vi "Create Data Clusters for Types.vi"(6 "Enum parameters":T1[](array[typedef]), 7 "Message parameters":T2[](array[typedef]), 8 "error in (no error)":errorcluster, 11 "Library in":refnum<vi>) -> (0 "error out":errorcluster, 3 "Library out":refnum<vi>)   [LabVIEW 2019, in "gRPC Template Creation Utility.lvlib"]
uses:
  gRPC Template Creation Utility.lvlib
  TypeDefs/Message Metadata (Scripting).ctl
  TypeDefs/Message Element Metadata (Scripting).ctl
  TypeDefs/Message Element Type.ctl
  TypeDefs/Enum Metadata (Scripting).ctl
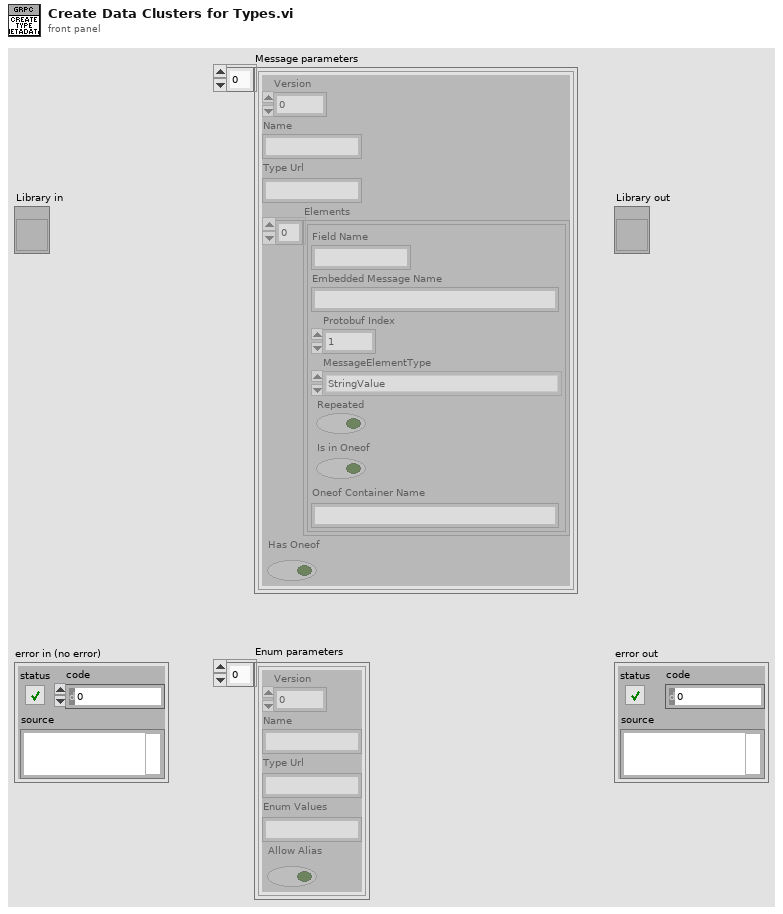
[diagram p1: front panel]
types:
  T1 = typedef "gRPC Template Creation Utility.lvlib/Enum Metadata (Scripting).ctl" = cluster{"Version":i32, "Name":string, "Type Url":string, "Enum Values":string, "Allow Alias":bool}
  T2 = typedef "gRPC Template Creation Utility.lvlib/Message Metadata (Scripting).ctl" = cluster{"Version":i32, "Name":string, "Type Url":string, "Elements":T3[], "Has Oneof":bool}
  T3 = typedef "gRPC Template Creation Utility.lvlib/Message Element Metadata (Scripting).ctl" = cluster{"Field Name":string, "Embedded Message Name":string, "Protobuf Index":i32, "MessageElementType":T4, "Repeated":bool, "Is in Oneof":bool, "Oneof Container Name":string}
  T4 = typedef "gRPC Template Creation Utility.lvlib/Message Element Type.ctl" = enum32{"Int32Value", "FloatValue", "DoubleValue", "BoolValue", "StringValue", "MessageValue", "Int64Value", "UInt32Value", "UInt64Value", "EnumValue", "Bytes", "Fixed64", "Fixed32", "SFixed64", "SFixed32", "SInt64", "SInt32"}
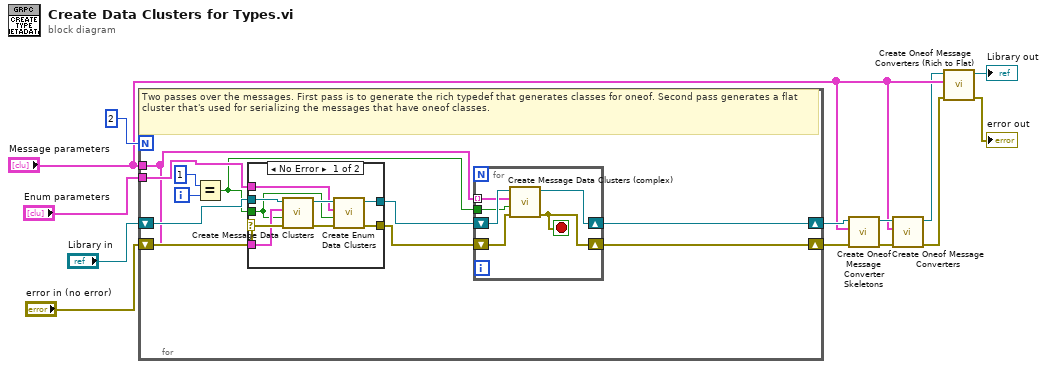
[diagram p0: block diagram]
diagram:
  n1 = for {
    N: 2 -> [_]
    tunnel: "Enum parameters" -> [w22]
    tunnel: "Message parameters" -> [w20]
    shift-right: [w18] -> w9
    shift-left: "Library in" -> [w24]
    shift-right: [w17] -> w8
    shift-left: "error in (no error)" -> [w23]
    i -> [w16]
    # "Two passes over the messages. First pass is to generate the rich typedef that generates classes for oneof. Second pass generates a flat cluster that's used for serializing the messages that have oneof classes."
    n2 = Equal?(x=1, y=w16) -> (x = y?=w14:bool)
    n3 = case shown="No Error" w23 {
      selector: w23 -> [w36 w40]
      tunnel: w20 -> [w33 _]
      tunnel: [w37 w41] -> w21
      tunnel: [w34 w40] -> w19
      tunnel: w24 -> [w39 w41]
      tunnel: w22 -> [w32 _]
      tunnel: w14 -> [w31 _]
      frame No Error {
        n4 = call "Create Message Data Clusters.vi"("error in (no error)"=w36, "Generate_SerializationHelper"=w31, "Message parameters"=w33, "Library"=w39) -> ("error out"=w35:errorcluster, "Library"=w38:refnum<vi>)  [unwired: 6 in]
        n5 = call "Create Enum Data Clusters.vi"("error in (no error)"=w35, "Generate_SerializationHelper"=w31, "Enum parameters"=w32, "Library in"=w38) -> ("error out"=w34:errorcluster, "Library out"=w37:refnum<vi>)  [unwired: 6 in]
      }
      frame Error {
      }
    }
    n6 = for {
      shift-right: [w28] -> w18
      shift-left: w21 -> [w30]
      shift-right: [w26] -> w17
      shift-left: w19 -> [w29]
      tunnel: w20 -> [w27] mode=indexing
      tunnel: w14 -> [w25]
      stop <- w26 stop-if-true
      n7 = call "Create Message Data Clusters (complex).vi"("error in (no error)"=w29, "Generate_SerializationHelper"=w25, "Message Metadata"=w27, "Library"=w30) -> ("error out"=w26:errorcluster, "Library"=w28:refnum<vi>)  [unwired: 6 in]
    }
  }
  n8 = call "Create Oneof Message Converter Skeletons.vi"("error in (no error)"=w8, "Message parameters"="Message parameters", "Library in"=w9) -> ("error out"=w7:errorcluster, "Library out"=w6:refnum<vi>)  [unwired: 7 in]
  n9 = call "Create Oneof Message Converters.vi"("error in (no error)"=w7, "Message parameters"="Message parameters", "Library in"=w6) -> ("error out"=w3:errorcluster, "Library out"=w4:refnum<vi>)  [unwired: 7 in]
  n10 = call "Create Oneof Message Converters (Rich to Flat).vi"("error in (no error)"=w3, "Message parameters"="Message parameters", "Library in"=w4) -> ("error out"=→"error out":errorcluster, "Library out"=→"Library out":refnum<vi>)  [unwired: 7 in]
